vi "Get OS Primary Language.vi"(8 "error in":errorcluster) -> (0 "error out":errorcluster, 1 "OS Primary Language":string)   [LabVIEW 2019]
doc: "Translates all VIs in registry list to the current language.\n\nTarget Language (current lang): Set this to update the current language and translate all VIs to this language. Do not wire to use the current language (If not set previously, thisi s by default the OS primary language)\n\nTo add VIs to the registry use the Register VI(s) function."
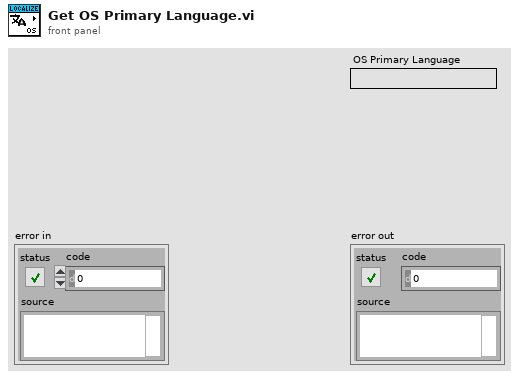
[diagram p1: front panel]
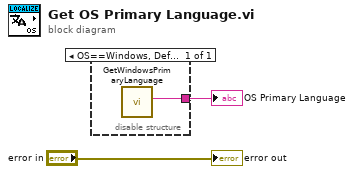
[diagram p0: block diagram]
diagram:
  n1 = disable-structure shown="OS==Windows, Default" {
    disable-tunnel: [w3] -> w2
    frame condition #0 (active) {
      n2 = call "GetWindowsPrimaryLanguage.vi"() -> ("Primary Language"=w3:string)  [unwired: 11 in]
    }
  }
  "OS Primary Language" <- w2
  "error out" <- "error in"
